vi "chaulin matador de porcos1.vi"() -> ()   [LabVIEW 2024]
uses:
  <vilib>/LabVIEW Open Source Project/Epoch Date & Time/epoch.UNIX/Epoch.UNIX.lvclass
panel:
  out "gráfico C":waveform(dbl)(graph)
  out "gráfico C":waveform(dbl)(graph)
  out "fase C":waveform(dbl)
  out "gráfico B":waveform(dbl)(graph)
  out "gráfico B":waveform(dbl)(graph)
  out "fase B":waveform(dbl)
  out "Gráfico A":waveform(dbl)(graph)
  out "gráfico A":waveform(dbl)(graph)
  in  "stop":bool
  out "fase A":waveform(dbl)
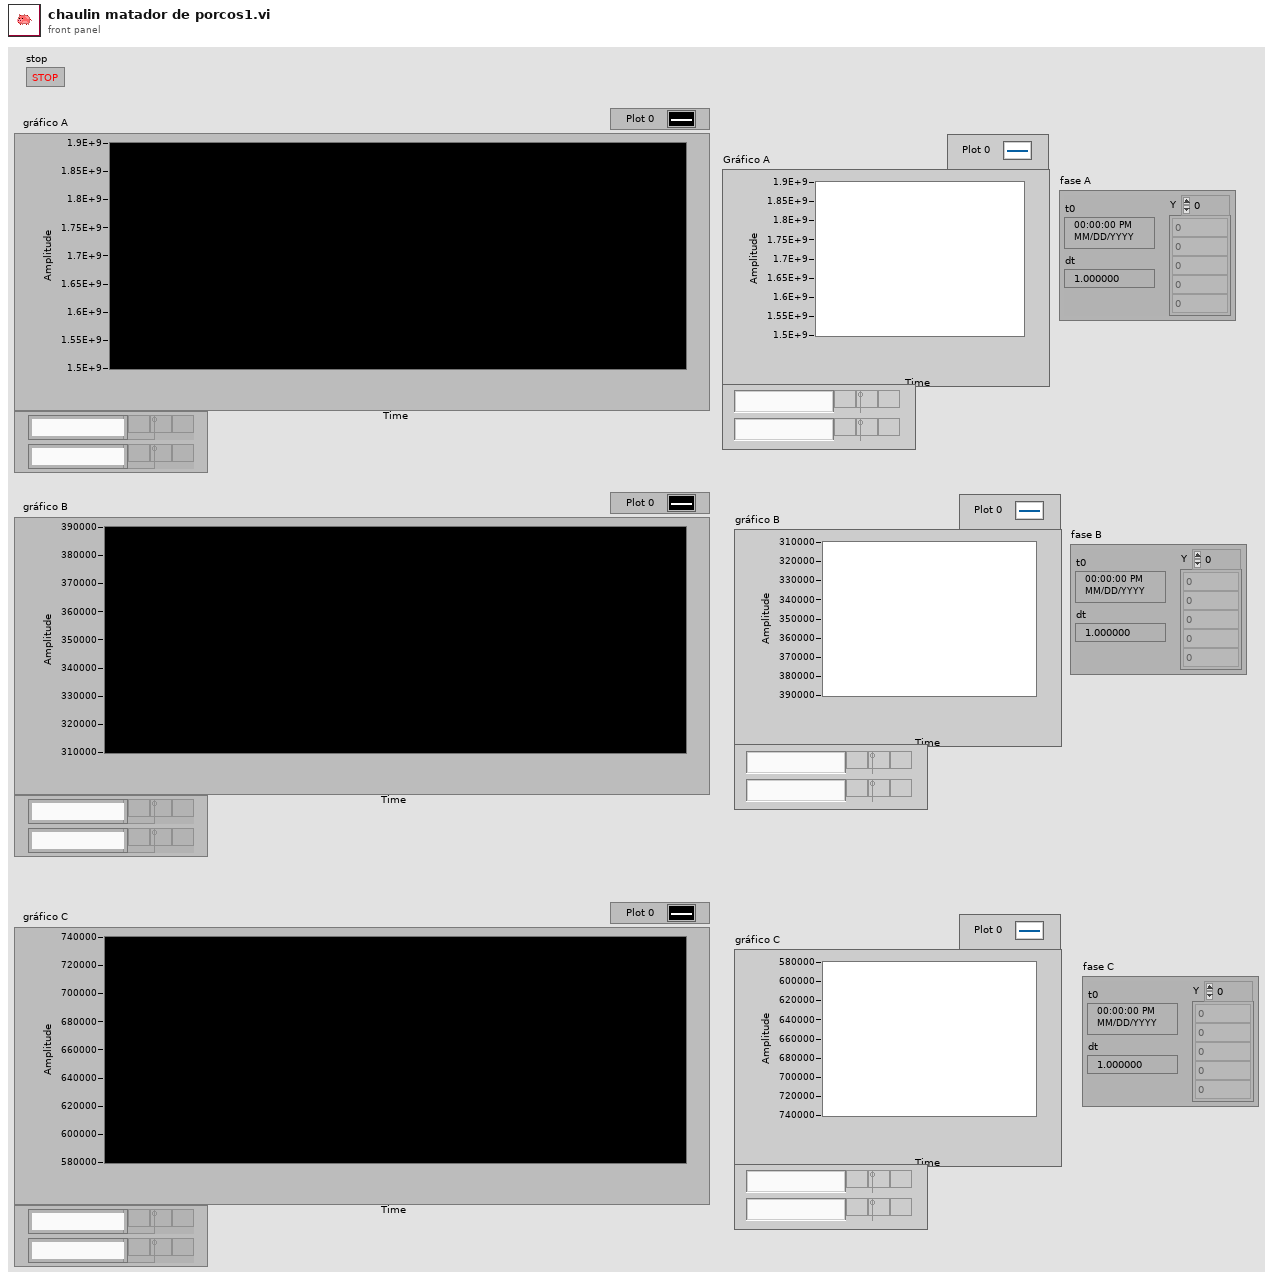
[diagram p1: front panel]
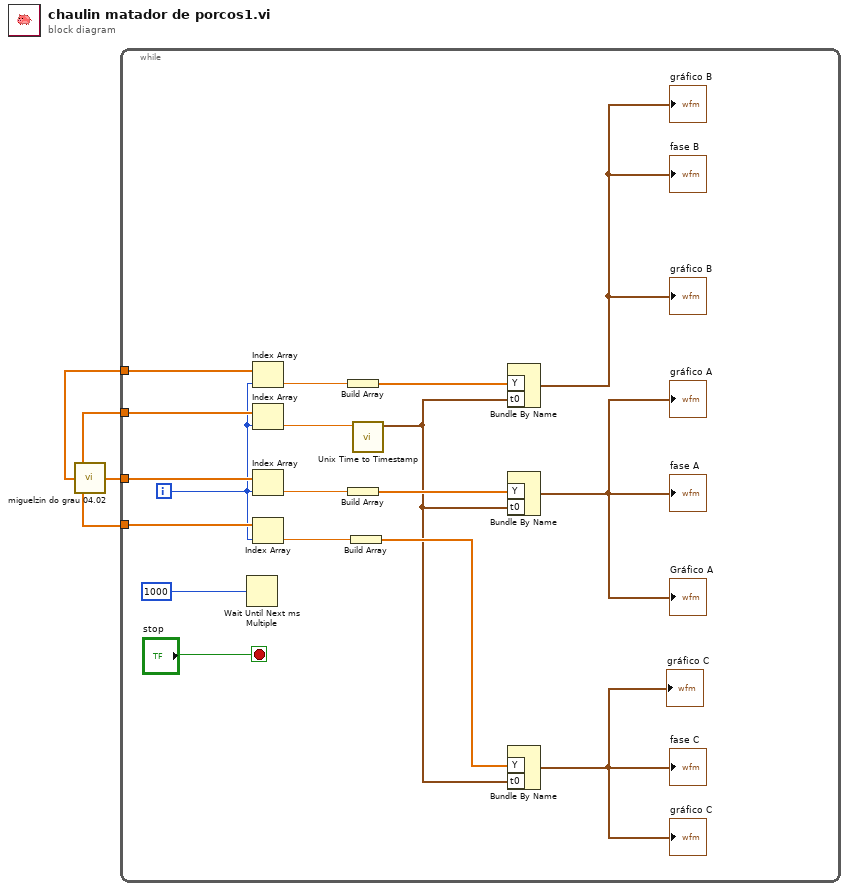
[diagram p0: block diagram]
diagram:
  n1 = call "miguelzin do grau 04.02.vi"() -> ("timestamp"=w3:dbl[], "C"=w1:dbl[], "B"=w2:dbl[], "A"=w4:dbl[])
  n2 = while {
    tunnel: w3 -> [w22]
    tunnel: w4 -> [w21]
    tunnel: w2 -> [w13]
    tunnel: w1 -> [w8]
    i -> [w5]
    stop <- "stop" stop-if-true
    n3 = Wait Until Next ms Multiple(millisecond multiple=u32 1000) -> ()  [unwired: 1 out]
    n4 = Index Array(array=w13, index=w5) -> (element=w12:dbl)
    n5 = Index Array(array=w21, index=w5) -> (element=w20:dbl)
    n6 = Index Array(array=w22, index=w5) -> (element=w17:dbl)
    n7 = Index Array(array=w8, index=w5) -> (element=w10:dbl)
    n8 = Build Array(w12) -> (w11:dbl[])
    n9 = Build Array(w17) -> (w18:dbl[])
    n10 = Build Array(w10) -> (w9:dbl[])
    n11 = call <vilib>:"Unix Time to Timestamp.vi"("Unix Time (s)"=w20) -> ("Timestamp"=w7:timestamp)  [unwired: 9 in, 1 out]
    n12 = Bundle By Name("Y"=w11, "t0"=w7) -> (→"fase B" →"gráfico B" →"gráfico B":waveform(dbl))  [unwired: 1 in]
    n13 = Bundle By Name("Y"=w18, "t0"=w7) -> (→"fase A" →"gráfico A" →"Gráfico A":waveform(dbl))  [unwired: 1 in]
    n14 = Bundle By Name("Y"=w9, "t0"=w7) -> (→"fase C" →"gráfico C" →"gráfico C":waveform(dbl))  [unwired: 1 in]
  }
